vi "main.vi"() -> ()   [LabVIEW 2015]
panel:
  out "error out":errorcluster
  in  "Controls":path
  in  "Library":path
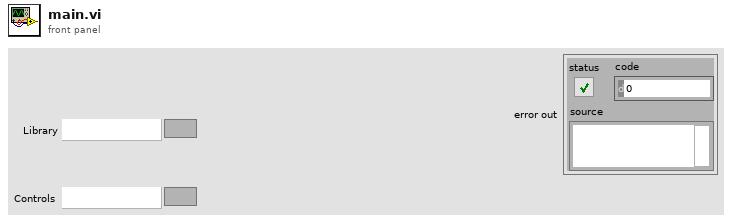
[diagram p1: front panel]
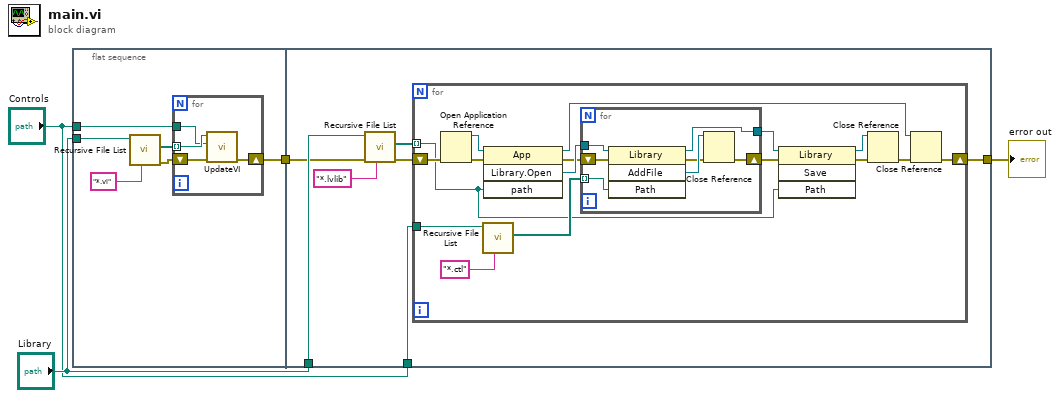
[diagram p0: block diagram]
diagram:
  n1 = flat-sequence {
    tunnel: "Controls" -> [w8]
    tunnel: "Library" -> [w5]
    tunnel: [w6] -> w4
    tunnel: w4 -> [w19]
    tunnel: "Library" -> [w20]
    tunnel: [w17] -> w2
    tunnel: "Controls" -> [w15]
    frame #0 {
      n2 = call <vilib>:"Recursive File List.vi"("pattern"="*.vi", "Folder Path"=w5) -> ("error out"=w7:errorcluster, "All Files in Dir"=w9:path[])  [unwired: 5 in, 3 out]
      n3 = for {
        tunnel: w9 -> [w14] mode=indexing
        tunnel: w8 -> [w13]
        shift-right: [w11] -> w6
        shift-left: w7 -> [w12]
        n4 = call "UpdateVI.vi"("error in (no error)"=w12, "Controls"=w13, "VIToUpdate"=w14) -> ("error out"=w11:errorcluster)  [unwired: 8 in]
      }
    }
    frame #1 {
      n5 = call <vilib>:"Recursive File List.vi"("pattern"="*.lvlib", "error in (no error)"=w19, "Folder Path"=w20) -> ("error out"=w18:errorcluster, "All Files in Dir"=w16:path[])  [unwired: 4 in, 3 out]
      n6 = for {
        shift-right: [w22] -> w17
        shift-left: w18 -> [w36]
        tunnel: w16 -> [w27] mode=indexing
        tunnel: w15 -> [w32]
        n7 = Open Application Reference(8:w36) -> (0:w35:errorcluster, 3:w37:refnum<vi>)  [unwired: 3 in]
        n8 = call <vilib>:"Recursive File List.vi"("pattern"="*.ctl", "Folder Path"=w32) -> ("All Files in Dir"=w31:path[])  [unwired: 5 in, 4 out]
        n9 = invoke class="App" method="Library.Open"(reference=w37, error in=w35, "path"=w27) -> (reference out=w23:refnum<vi>, error out=w30:errorcluster, "Open Library"=w34:refnum<vi>)  [unwired: 1 in, 1 out]
        n10 = for {
          tunnel: w34 -> [w44]
          tunnel: w31 -> [w43] mode=indexing
          shift-right: [w39] -> w28
          shift-left: w30 -> [w42]
          tunnel: [w38] -> w29
          n11 = invoke class="Library" method="AddFile"(reference=w44, error in=w42, "Path"=w43) -> (reference out=w38:refnum<vi>, error out=w40:errorcluster, "AddFile"=w41:refnum<vi>)  [unwired: 1 in, 1 out]
          n12 = Close Reference(reference=w41, error in (no error)=w40) -> (error out=w39:errorcluster)
        }
        n13 = invoke class="Library" method="Save"(reference=w29, error in=w28, "Path"=w27) -> (reference out=w25:refnum<vi>, error out=w26:errorcluster)  [unwired: 1 in, 2 out]
        n14 = Close Reference(reference=w25, error in (no error)=w26) -> (error out=w24:errorcluster)
        n15 = Close Reference(reference=w23, error in (no error)=w24) -> (error out=w22:errorcluster)
      }
    }
  }
  "error out" <- w2
